vi "_Test_main.vi"() -> ()   [LabVIEW 2017]
uses:
  _Typedef/Def-IniSettings -- Cluster.ctl
panel:
  in  "stop":bool
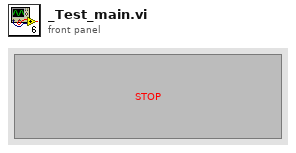
[diagram p1: front panel]
types:
  T1 = typedef "Def-IniSettings -- Cluster.ctl" = cluster{"address":string, "receiver port":u16, "Ignore Gateway IP":bool, "HostName":string}
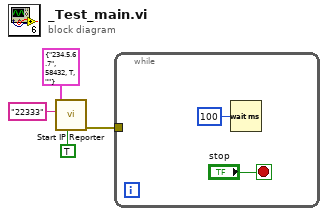
[diagram p0: block diagram]
diagram:
  n1 = call "Start IP Reporter.vi"("Load From File(F)"=TRUE, "Information"="22333", "Setttings"=T1 {"address"="234.5.6.7", "receiver port"=58432, "Ignore Gateway IP"=TRUE, "HostName"=""}) -> ("error out"=w3:errorcluster)  [unwired: 8 in]
  n2 = while {
    tunnel: w3 -> [_]
    stop <- "stop" stop-if-true
    n3 = Wait (ms)(milliseconds to wait=u32 100) -> ()  [unwired: 1 out]
  }
